vi "filter.filter.other.vi"(11 "filter.data in":T1 {"memory.command"."order.slot.value"."Quantity" format="%016x"; "memory.command"."order.slot.value"."OrderId" format="%016x"; "memory.command"."ticker.slot.value"."Symbol" format="%016x"; "Scratch"."OrderId" format="%016x"}) -> (3 "filter.data out":T1 {"memory.command"."order.slot.value"."Quantity" format="%016x"; "memory.command"."order.slot.value"."OrderId" format="%016x"; "memory.command"."ticker.slot.value"."Symbol" format="%016x"; "Scratch"."OrderId" format="%016x"})   [LabVIEW 2022 SP3]
uses:
  filter.data.ctl
  filter.states.ctl
  filter.debug.ctl
  filter.debug.slot.ctl
  filter.data.scratch.ctl
  common/orderbook.command.ctl
  common/orderbook.command.type.ctl
  filter.memory.command.ctl
  ticker.slot.ctl
  order.slot.ctl
  filter.getstate.ctl
  filter.getstate.slot.ctl
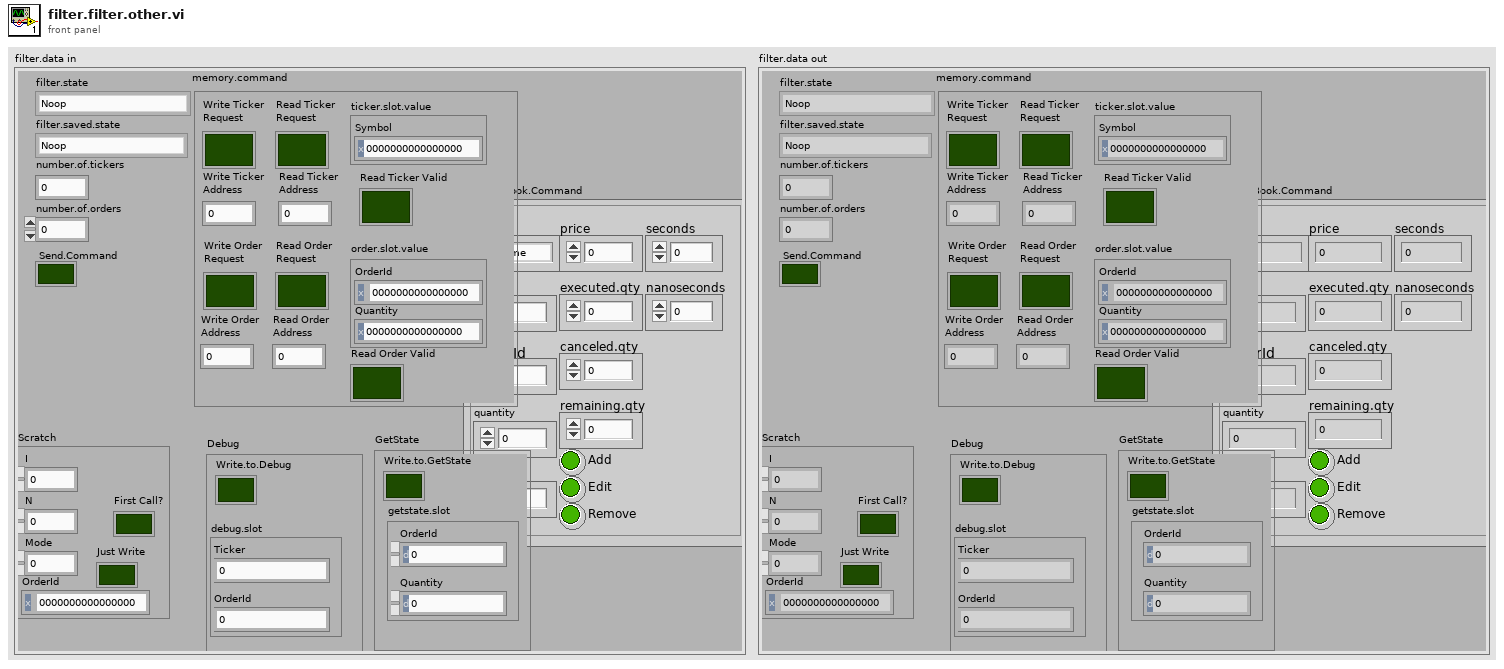
[diagram p1: front panel]
types:
  T1 = typedef "filter.data.ctl" = cluster{"filter.state":T2, "Debug":T3, "number.of.tickers":u32, "number.of.orders":u32, "filter.saved.state":T2, "Scratch":T5, "OrderBook.Command":T6, "Send.Command":bool, "memory.command":T8, "GetState":T11}
  T2 = typedef "filter.states.ctl" = enum16{"Noop", "Reset", "Debug", "Configuration", "Get.State", "Wait.for.Command", "Filter.Add", "Filter.Other", "Insert.Order", "Delete Order"}
  T3 = typedef "filter.debug.ctl" = cluster{"Write.to.Debug":bool, "debug.slot":T4}
  T4 = typedef "filter.debug.slot.ctl" = cluster{"Ticker":u64, "OrderId":u64}
  T5 = typedef "filter.data.scratch.ctl" = cluster{"I":u32, "N":u32, "Mode":u32, "OrderId":u64, "First Call?":bool, "Just Write":bool}
  T6 = typedef "orderbook.command.ctl" = cluster{"type":T7, "side":u8, "orderId ":u64, "quantity":u32, "symbol":u64, "price":u64, "executed.qty":u32, "canceled.qty":u32, "remaining.qty":u32, "seconds":u64, "nanoseconds":u64, "Add":bool, "Edit":bool, "Remove":bool}
  T7 = typedef "orderbook.command.type.ctl" = enum8{"Time", "AddOrder", "OrderExecuted", "OrderExecutedAtPrice", "ReduceSize", "ModifyOrder", "DeleteOrder", "Get.Everything", "Get.All.Orders", "Get.Top"}
  T8 = typedef "filter.memory.command.ctl" = cluster{"ticker.slot.value":T9, "order.slot.value":T10, "Write Ticker\nAddress":u32, "Write Ticker\nRequest":bool, "Read Ticker\nRequest":bool, "Read Ticker\nAddress":u32, "Read Ticker Valid":bool, "Write Order\nAddress":u32, "Write Order\nRequest":bool, "Read Order\nRequest":bool, "Read Order\nAddress":u32, "Read Order Valid":bool}
  T9 = typedef "ticker.slot.ctl" = cluster{"Symbol":u64}
  T10 = typedef "order.slot.ctl" = cluster{"OrderId":u64, "Quantity":u64}
  T11 = typedef "filter.getstate.ctl" = cluster{"Write.to.GetState":bool, "getstate.slot":T12}
  T12 = typedef "filter.getstate.slot.ctl" = cluster{"OrderId":u64, "Quantity":u64}
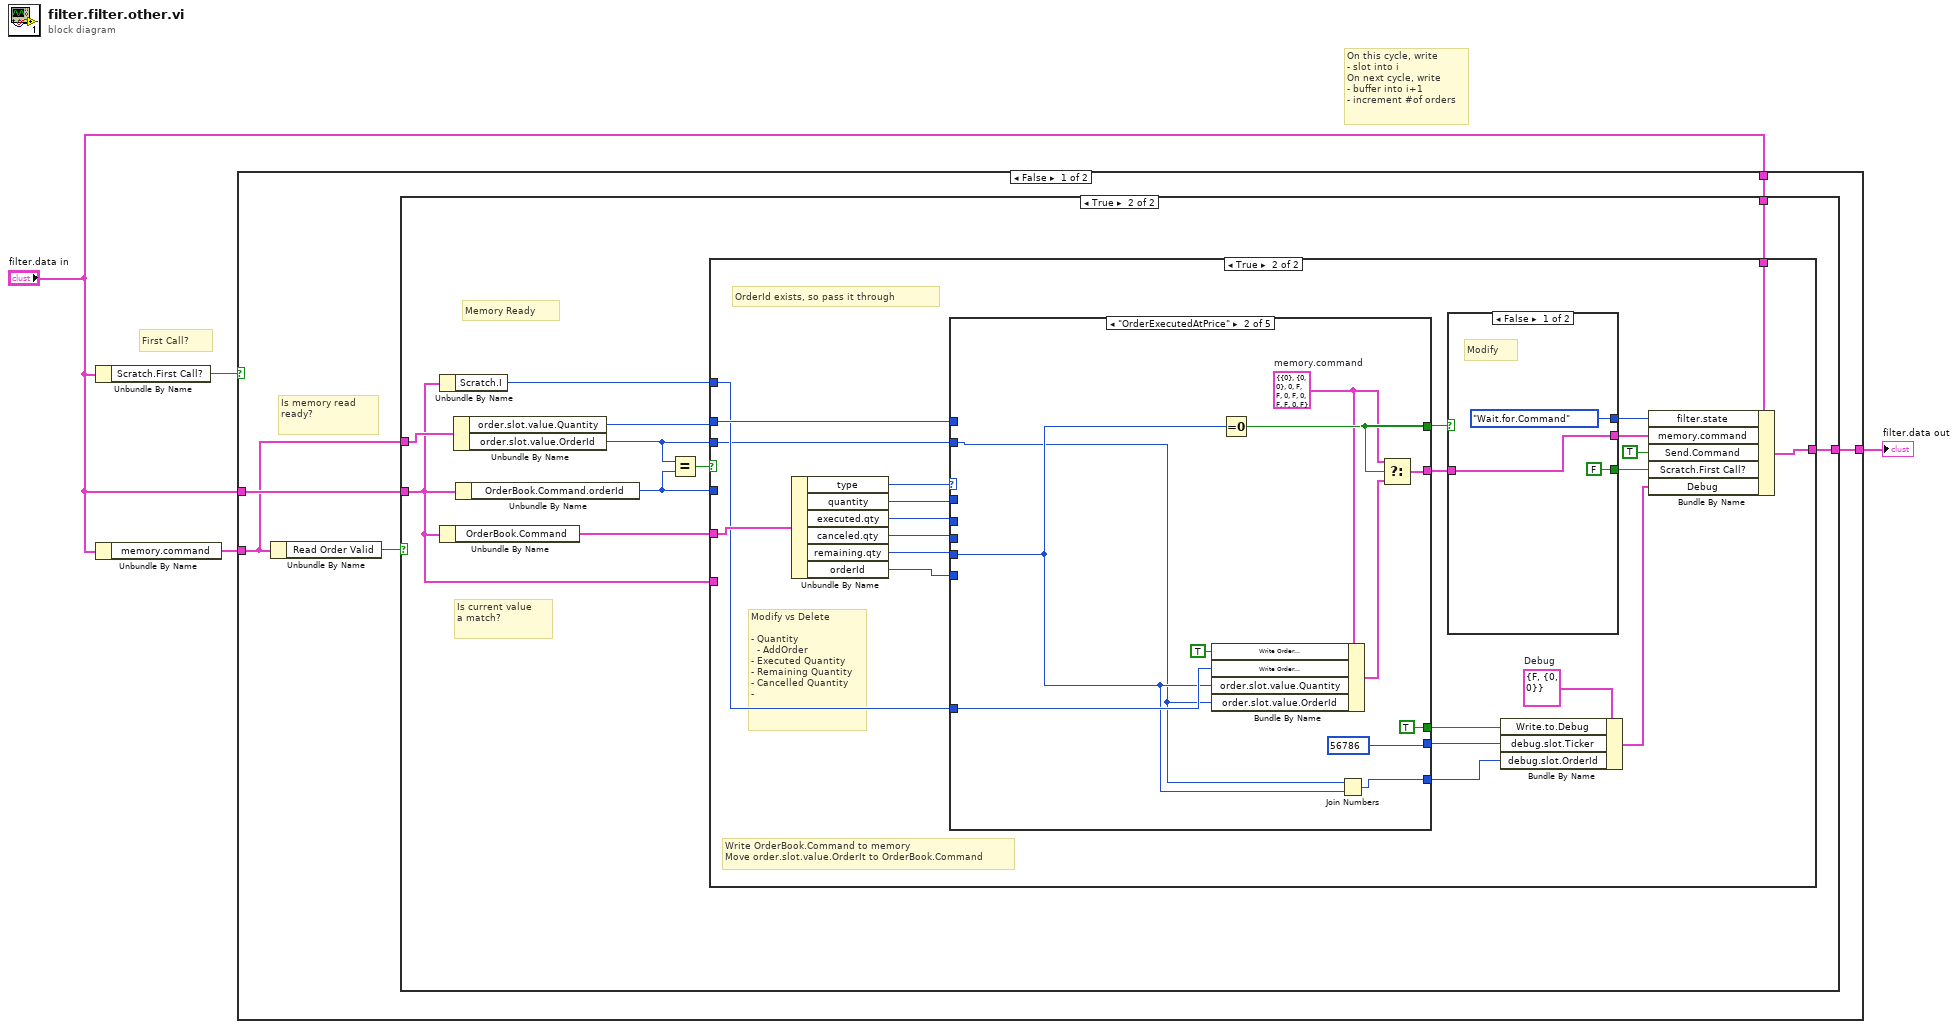
[diagram p0: block diagram]
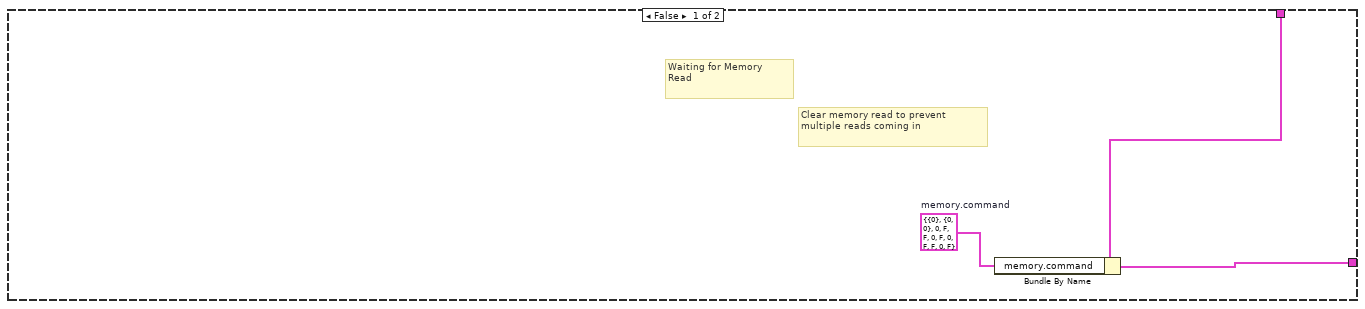
[diagram p2: hidden frame]
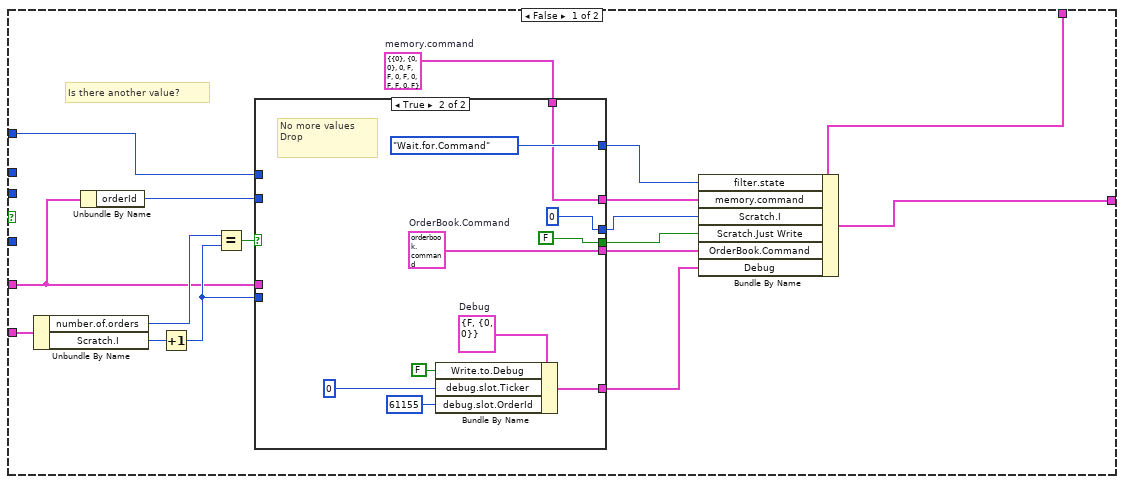
[diagram p3: hidden frame]
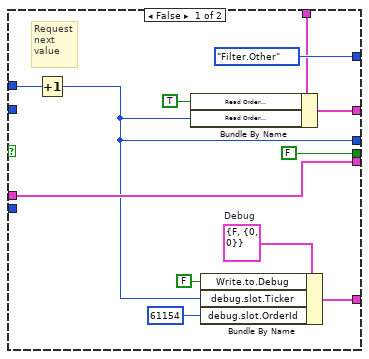
[diagram p4: hidden frame]
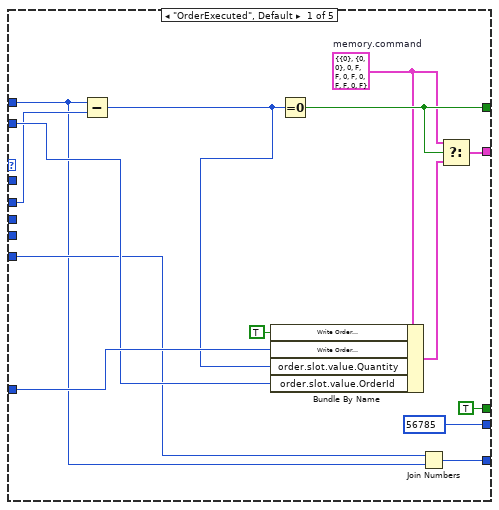
[diagram p5: hidden frame]
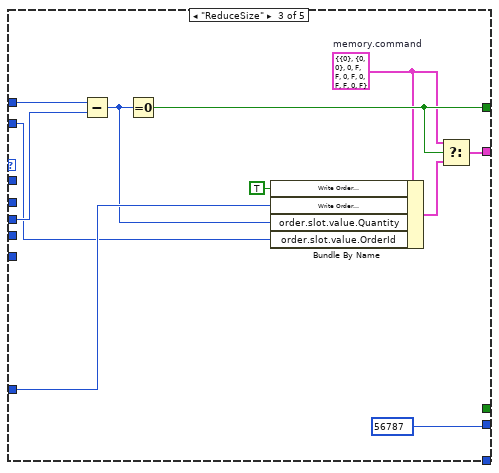
[diagram p6: hidden frame]
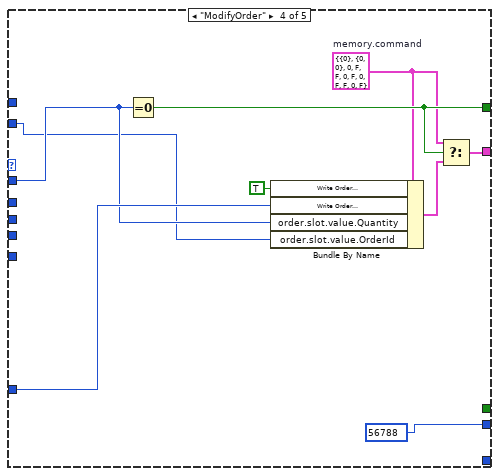
[diagram p7: hidden frame]
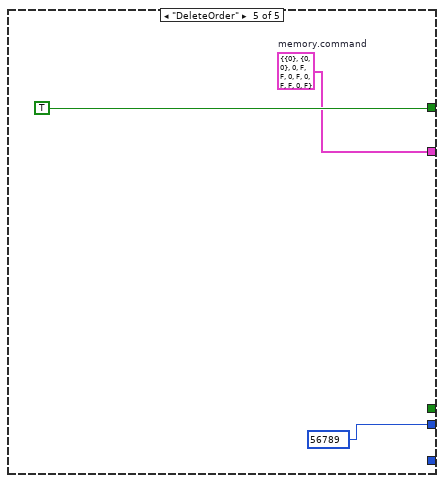
[diagram p8: hidden frame]
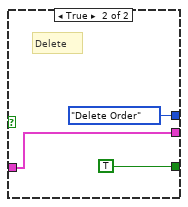
[diagram p9: hidden frame]
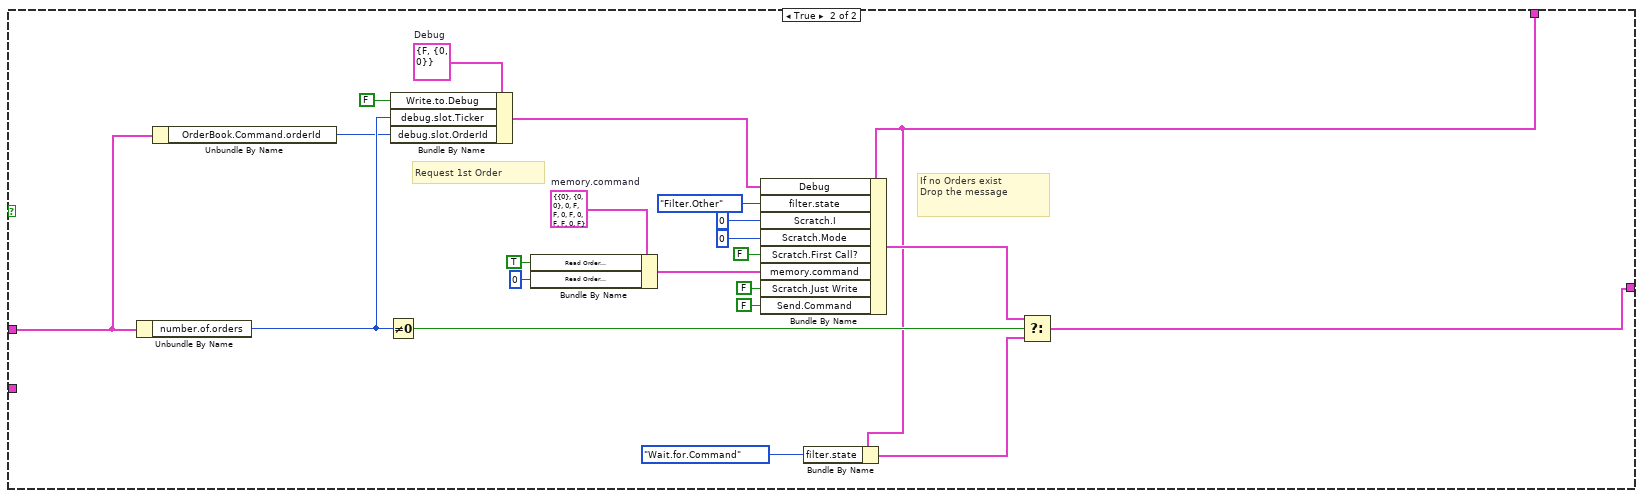
[diagram p10: hidden frame]
diagram:
  # "On this cycle, write\n- slot into i\nOn next cycle, write\n- buffer into i+1\n- increment #of orders"
  # "First Call?"
  n1 = Unbundle By Name("filter.data in") -> ("Scratch.First Call?"=w1:bool)
  n2 = Unbundle By Name("filter.data in") -> ("memory.command"=w3:T8)
  n3 = case shown="False" w1 {
    tunnel: "filter.data in" -> [w8 w140]
    tunnel: [w9 w141] -> w2
    tunnel: w3 -> [w6 _]
    tunnel: "filter.data in" -> [w7 w142]
    frame False {
      # "Is memory read\nready?"
      n4 = Unbundle By Name(w6) -> ("Read Order Valid"=w5:bool)
      n5 = case shown="True" w5 {
        tunnel: [w10 w20] -> w9
        tunnel: w8 -> [w12 w21]
        tunnel: w7 -> [_ w19]
        tunnel: w6 -> [_ w22]
        frame False {
          w11 = T8 {"ticker.slot.value"={"Symbol"=0}, "order.slot.value"={"OrderId"=0, "Quantity"=0}, "Write Ticker\nAddress"=0, "Write Ticker\nRequest"=FALSE, "Read Ticker\nRequest"=FALSE, "Read Ticker\nAddress"=0, "Read Ticker Valid"=FALSE, "Write Order\nAddress"=0, "Write Order\nRequest"=FALSE, "Read Order\nRequest"=FALSE, "Read Order\nAddress"=0, "Read Order Valid"=FALSE}  # memory.command
          # "Clear memory read to prevent\nmultiple reads coming in"
          # "Waiting for Memory\nRead"
          n6 = Bundle By Name(cluster=w12, "memory.command"=w11) -> (w10:T1)
        }
        frame True {
          # "Is current value\na match?"
          # "Memory Ready"
          n7 = Unbundle By Name(w19) -> ("Scratch.I"=w14:u32)
          n8 = Unbundle By Name(w19) -> ("OrderBook.Command"=w17:T6)
          n9 = Unbundle By Name(w22) -> ("order.slot.value.Quantity"=w13:u64, "order.slot.value.OrderId"=w16:u64)
          n10 = Unbundle By Name(w19) -> ("OrderBook.Command.orderId"=w15:u64)
          n11 = Equal?(x=w16, y=w15) -> (x = y?=w18:bool)
          n12 = case shown="True" w18 {
            tunnel: w21 -> [w38 w84]
            tunnel: [w39 w82] -> w20
            tunnel: w17 -> [w24 w81]
            tunnel: w19 -> [w37 _]
            tunnel: w16 -> [_ w66]
            tunnel: w14 -> [w29 w73]
            tunnel: w15 -> [_ _]
            tunnel: w13 -> [_ w77]
            frame False {
              w31 = T8 {"ticker.slot.value"={"Symbol"=0}, "order.slot.value"={"OrderId"=0, "Quantity"=0}, "Write Ticker\nAddress"=0, "Write Ticker\nRequest"=FALSE, "Read Ticker\nRequest"=FALSE, "Read Ticker\nAddress"=0, "Read Ticker Valid"=FALSE, "Write Order\nAddress"=0, "Write Order\nRequest"=FALSE, "Read Order\nRequest"=FALSE, "Read Order\nAddress"=0, "Read Order Valid"=FALSE}  # memory.command
              # "Is there another value?"
              n13 = Unbundle By Name(w37) -> ("number.of.orders"=w28:u32, "Scratch.I"=w36:u32)
              n14 = Unbundle By Name(w24) -> ("orderId"=w30:u64)
              n15 = Increment(x=w36) -> (x+1=w33:u32)
              n16 = Equal?(x=w28, y=w33) -> (x = y?=w34:bool)
              n17 = case shown="True" w34 {
                tunnel: [w51 w53] -> w35
                tunnel: w33 -> [_ _]
                tunnel: [filter.states."Filter.Other" ("filter.state") filter.states."Wait.for.Command" ("filter.state")] -> w32
                tunnel: w31 -> [w48 w53]
                tunnel: w30 -> [_ _]
                tunnel: w29 -> [w41 _]
                tunnel: [w40 u32 0] -> w27
                tunnel: [FALSE ("Scratch.Just Write") FALSE ("Scratch.Just Write")] -> w26
                tunnel: [w46 w58] -> w25
                tunnel: w24 -> [w46 _]
                tunnel: [w44 w56] -> w23
                frame False {
                  w45 = T3 {"Write.to.Debug"=FALSE, "debug.slot"={"Ticker"=0, "OrderId"=0}}  # Debug
                  # "Request\nnext\nvalue"
                  n18 = Increment(x=w41) -> (x+1=w40:u32)
                  n19 = Bundle By Name(cluster=w48, "Read Order\nRequest"=TRUE ("Read.Request"), "Read Order\nAddress"=w40) -> (w51:T8)
                  n20 = Bundle By Name(cluster=w45, "Write.to.Debug"=FALSE, "debug.slot.Ticker"=w40, "debug.slot.OrderId"=u64 61154) -> (w44:T3)
                }
                frame True {
                  w57 = T3 {"Write.to.Debug"=FALSE, "debug.slot"={"Ticker"=0, "OrderId"=0}}  # Debug
                  w58 = T6 {"type"=enum."Time", "side"=0, "orderId "=0, "quantity"=0, "symbol"=0, "price"=0, "executed.qty"=0, "canceled.qty"=0, "remaining.qty"=0, "seconds"=0, "nanoseconds"=0, "Add"=FALSE, "Edit"=FALSE, "Remove"=FALSE}  # OrderBook.Command
                  # "No more values\nDrop"
                  n21 = Bundle By Name(cluster=w57, "Write.to.Debug"=FALSE, "debug.slot.Ticker"=u64 0, "debug.slot.OrderId"=u64 61155) -> (w56:T3)
                }
              }
              n22 = Bundle By Name(cluster=w38, "filter.state"=w32, "memory.command"=w35, "Scratch.I"=w27, "Scratch.Just Write"=w26, "OrderBook.Command"=w25, "Debug"=w23) -> (w39:T1)
            }
            frame True {
              w79 = T3 {"Write.to.Debug"=FALSE, "debug.slot"={"Ticker"=0, "OrderId"=0}}  # Debug
              # "Modify vs Delete\n\n- Quantity\n  - AddOrder\n- Executed Quantity\n- Remaining Quantity\n- Cancelled Quantity\n-"
              # "Write OrderBook.Command to memory\nMove order.slot.value.OrderIt to OrderBook.Command"
              # "OrderId exists, so pass it through"
              n23 = Unbundle By Name(w81) -> ("type"=w78:T7, "quantity"=w72:u32, "executed.qty"=w69:u32, "canceled.qty"=w70:u32, "remaining.qty"=w71:u32, "orderId"=w65:u64)
              n24 = case shown="\"OrderExecutedAtPrice\"" w78 {
                tunnel: w77 -> [w86 _ w120 _ _]
                tunnel: w72 -> [_ _ _ w123 _]
                tunnel: [w97 w108 w118 w128 TRUE] -> w76
                tunnel: [w95 w106 w116 w126 w131] -> w75
                tunnel: w73 -> [w93 w104 w114 w124 _]
                tunnel: w71 -> [_ w101 _ _ _]
                tunnel: w70 -> [_ _ w112 _ _]
                tunnel: w69 -> [w87 _ _ _ _]
                tunnel: [TRUE ("Write.to.Debug") TRUE ("Write.to.Debug") _ _ _] -> w68
                tunnel: [w89 w102 _ _ _] -> w67
                tunnel: w66 -> [w91 w99 w111 w122 _]
                tunnel: w65 -> [w90 _ _ _ _]
                tunnel: [u64 56785 ("debug.slot.Ticker") u64 56786 ("debug.slot.Ticker") u64 56787 ("debug.slot.Ticker") u64 56788 ("debug.slot.Ticker") u64 56789 ("debug.slot.Ticker")] -> w62
                frame "OrderExecuted", Default {
                  w94 = T8 {"ticker.slot.value"={"Symbol"=0}, "order.slot.value"={"OrderId"=0, "Quantity"=0}, "Write Ticker\nAddress"=0, "Write Ticker\nRequest"=FALSE, "Read Ticker\nRequest"=FALSE, "Read Ticker\nAddress"=0, "Read Ticker Valid"=FALSE, "Write Order\nAddress"=0, "Write Order\nRequest"=FALSE, "Read Order\nRequest"=FALSE, "Read Order\nAddress"=0, "Read Order Valid"=FALSE}  # memory.command
                  n25 = Subtract(x=w86, y=w87) -> (x-y=w88:u64)
                  n26 = Bundle By Name(cluster=w94, "Write Order\nRequest"=TRUE ("Read.Request"), "Write Order\nAddress"=w93, "order.slot.value.Quantity"=w88, "order.slot.value.OrderId"=w91) -> (w96:T8)
                  n27 = Equal To 0?(x=w88) -> (x = 0?=w97:bool)
                  n28 = Join Numbers(hi=w90, lo=w86) -> ((hi.lo)=w89:u64)
                  n29 = Select(t=w94, s=w97, f=w96) -> (s? t:f=w95:T8)
                }
                frame "OrderExecutedAtPrice" {
                  w105 = T8 {"ticker.slot.value"={"Symbol"=0}, "order.slot.value"={"OrderId"=0, "Quantity"=0}, "Write Ticker\nAddress"=0, "Write Ticker\nRequest"=FALSE, "Read Ticker\nRequest"=FALSE, "Read Ticker\nAddress"=0, "Read Ticker Valid"=FALSE, "Write Order\nAddress"=0, "Write Order\nRequest"=FALSE, "Read Order\nRequest"=FALSE, "Read Order\nAddress"=0, "Read Order Valid"=FALSE}  # memory.command
                  n30 = Bundle By Name(cluster=w105, "Write Order\nRequest"=TRUE ("Read.Request"), "Write Order\nAddress"=w104, "order.slot.value.Quantity"=w101, "order.slot.value.OrderId"=w99) -> (w107:T8)
                  n31 = Equal To 0?(x=w101) -> (x = 0?=w108:bool)
                  n32 = Join Numbers(hi=w99, lo=w101) -> ((hi.lo)=w102:u64)
                  n33 = Select(t=w105, s=w108, f=w107) -> (s? t:f=w106:T8)
                }
                frame "ReduceSize" {
                  w115 = T8 {"ticker.slot.value"={"Symbol"=0}, "order.slot.value"={"OrderId"=0, "Quantity"=0}, "Write Ticker\nAddress"=0, "Write Ticker\nRequest"=FALSE, "Read Ticker\nRequest"=FALSE, "Read Ticker\nAddress"=0, "Read Ticker Valid"=FALSE, "Write Order\nAddress"=0, "Write Order\nRequest"=FALSE, "Read Order\nRequest"=FALSE, "Read Order\nAddress"=0, "Read Order Valid"=FALSE}  # memory.command
                  n34 = Subtract(x=w120, y=w112) -> (x-y=w113:u64)
                  n35 = Equal To 0?(x=w113) -> (x = 0?=w118:bool)
                  n36 = Bundle By Name(cluster=w115, "Write Order\nRequest"=TRUE ("Read.Request"), "Write Order\nAddress"=w114, "order.slot.value.Quantity"=w113, "order.slot.value.OrderId"=w111) -> (w117:T8)
                  n37 = Select(t=w115, s=w118, f=w117) -> (s? t:f=w116:T8)
                }
                frame "ModifyOrder" {
                  w125 = T8 {"ticker.slot.value"={"Symbol"=0}, "order.slot.value"={"OrderId"=0, "Quantity"=0}, "Write Ticker\nAddress"=0, "Write Ticker\nRequest"=FALSE, "Read Ticker\nRequest"=FALSE, "Read Ticker\nAddress"=0, "Read Ticker Valid"=FALSE, "Write Order\nAddress"=0, "Write Order\nRequest"=FALSE, "Read Order\nRequest"=FALSE, "Read Order\nAddress"=0, "Read Order Valid"=FALSE}  # memory.command
                  n38 = Equal To 0?(x=w123) -> (x = 0?=w128:bool)
                  n39 = Bundle By Name(cluster=w125, "Write Order\nRequest"=TRUE ("Read.Request"), "Write Order\nAddress"=w124, "order.slot.value.Quantity"=w123, "order.slot.value.OrderId"=w122) -> (w127:T8)
                  n40 = Select(t=w125, s=w128, f=w127) -> (s? t:f=w126:T8)
                }
                frame "DeleteOrder" {
                  w131 = T8 {"ticker.slot.value"={"Symbol"=0}, "order.slot.value"={"OrderId"=0, "Quantity"=0}, "Write Ticker\nAddress"=0, "Write Ticker\nRequest"=FALSE, "Read Ticker\nRequest"=FALSE, "Read Ticker\nAddress"=0, "Read Ticker Valid"=FALSE, "Write Order\nAddress"=0, "Write Order\nRequest"=FALSE, "Read Order\nRequest"=FALSE, "Read Order\nAddress"=0, "Read Order Valid"=FALSE}  # memory.command
                }
              }
              n41 = case shown="False" w76 {
                tunnel: [filter.states."Wait.for.Command" ("filter.state") filter.states."Delete Order" ("filter.state")] -> w83
                tunnel: [w134 w137] -> w74
                tunnel: w75 -> [w134 w137]
                tunnel: [FALSE TRUE] -> w63
                frame False {
                  # "Modify"
                }
                frame True {
                  # "Delete"
                }
              }
              n42 = Bundle By Name(cluster=w79, "Write.to.Debug"=w68, "debug.slot.Ticker"=w62, "debug.slot.OrderId"=w67) -> (w64:T3)
              n43 = Bundle By Name(cluster=w84, "filter.state"=w83, "memory.command"=w74, "Send.Command"=TRUE, "Scratch.First Call?"=w63, "Debug"=w64) -> (w82:T1)
            }
          }
        }
      }
    }
    frame True {
      w149 = T3 {"Write.to.Debug"=FALSE, "debug.slot"={"Ticker"=0, "OrderId"=0}}  # Debug
      w159 = T8 {"ticker.slot.value"={"Symbol"=0}, "order.slot.value"={"OrderId"=0, "Quantity"=0}, "Write Ticker\nAddress"=0, "Write Ticker\nRequest"=FALSE, "Read Ticker\nRequest"=FALSE, "Read Ticker\nAddress"=0, "Read Ticker Valid"=FALSE, "Write Order\nAddress"=0, "Write Order\nRequest"=FALSE, "Read Order\nRequest"=FALSE, "Read Order\nAddress"=0, "Read Order Valid"=FALSE}  # memory.command
      # "If no Orders exist\nDrop the message"
      # "Request 1st Order"
      n44 = Unbundle By Name(w142) -> ("number.of.orders"=w146:u32)
      n45 = Unbundle By Name(w142) -> ("OrderBook.Command.orderId"=w145:u64)
      n46 = Not Equal To 0?(x=w146) -> (x != 0?=w144:bool)
      n47 = Bundle By Name(cluster=w149, "Write.to.Debug"=FALSE, "debug.slot.Ticker"=w146, "debug.slot.OrderId"=w145) -> (w147:T3)
      n48 = Bundle By Name(cluster=w159, "Read Order\nRequest"=TRUE ("Read.Request"), "Read Order\nAddress"=u32 0 ("Read Order\nAddress")) -> (w154:T8)
      n49 = Bundle By Name(cluster=w140, "Debug"=w147, "filter.state"=filter.states."Filter.Other", "Scratch.I"=u32 0, "Scratch.Mode"=u32 0, "Scratch.First Call?"=FALSE, "memory.command"=w154, "Scratch.Just Write"=FALSE, "Send.Command"=FALSE) -> (w153:T1)
      n50 = Bundle By Name(cluster=w140, "filter.state"=filter.states."Wait.for.Command") -> (w152:T1)
      n51 = Select(t=w153, s=w144, f=w152) -> (s? t:f=w141:T1)
    }
  }
  "filter.data out" <- w2
